vi "UpdateSelectedData.vi"(8 "error in (no error)":errorcluster, 9 "Old Value":i32, 11 "FakedArray in":refnum<class "FakedArray.lvclass">) -> (0 "error out":errorcluster, 3 "FakedArray out":refnum<class "FakedArray.lvclass">)   [LabVIEW 2020, in "FakedArray.lvclass"]
uses:
  FakedArray.lvclass
  FakedArray.lvclass/FakedArray.ctl
  vi.lib/LabVIEW Icon API/lv_icon/Controls/IEColor.ctl
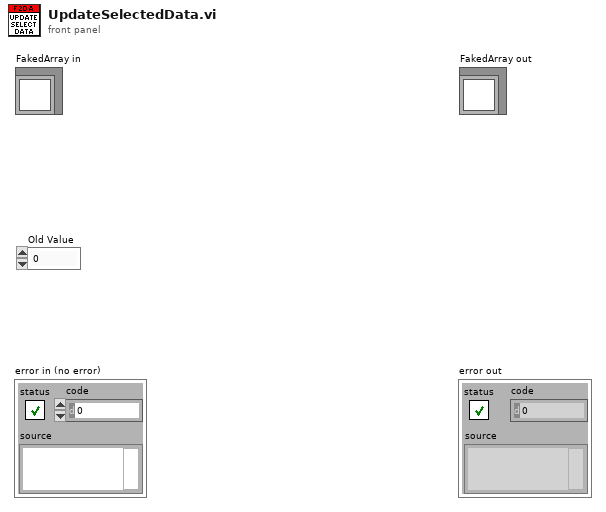
[diagram p1: front panel]
types:
  T1 = typedef "IEColor.ctl" = u32
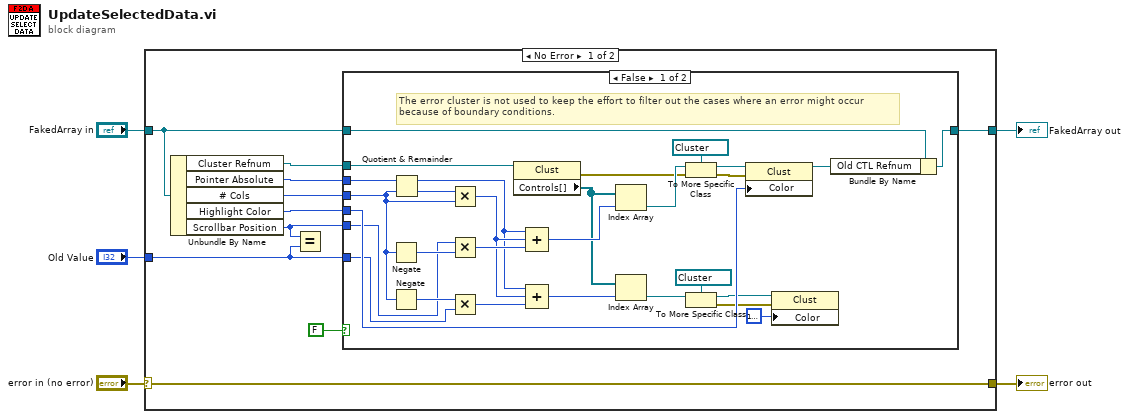
[diagram p0: block diagram]
diagram:
  n1 = case shown="No Error" "error in (no error)" {
    selector: "error in (no error)" -> [w7 w47]
    tunnel: [w7 w47] -> w4
    tunnel: [w10 w46] -> w2
    tunnel: "FakedArray in" -> [w15 w46]
    tunnel: "Old Value" -> [w8 _]
    frame No Error {
      n2 = Unbundle By Name(w15) -> ("Cluster Refnum"=w13:refnum<vi>, "Pointer Absolute"=w14:i32, "# Cols"=w11:i32, "Highlight Color"=w12:T1, "Scrollbar Position"=w9:i32)
      n3 = Equal?(x=w9, y=w8) -> ()  [unwired: 1 out]
      n4 = case shown="False" FALSE {
        tunnel: w15 -> [w44 w45]
        tunnel: w14 -> [w43 _]
        tunnel: w13 -> [w41 _]
        tunnel: w12 -> [w35 _]
        tunnel: w11 -> [w30 _]
        tunnel: [w19 w45] -> w10
        tunnel: w9 -> [w17 _]
        tunnel: w8 -> [w16 _]
        frame False {
          # "The error cluster is not used to keep the effort to filter out the cases where an error might occur\nbecause of boundary conditions."
          n5 = Negate(x=w30) -> (-x=w31:i32)
          n6 = Negate(x=w30) -> (-x=w32:i32)
          n7 = Quotient & Remainder(x=w43, y=w30) -> (x-y*floor(x/y)=w27:i32, floor(x/y)=w42:i32)
          n8 = Multiply(x=w42, y=w30) -> (x*y=w28:i32)
          n9 = Multiply(x=w17, y=w31) -> (x*y=w34:i32)
          n10 = Multiply(x=w32, y=w16) -> (x*y=w29:i32)
          n11 = property class="Clust"(reference=w41) -> (error out=w38:errorcluster, "Controls[]"=w26:refnum<vi>[])  [unwired: 1 in, 1 out]
          n12 = Compound Arithmetic op=ADD(w27, w28, w34) -> (w33:i32)
          n13 = Compound Arithmetic op=ADD(w27, w28, w29) -> (w25:i32)
          n14 = Index Array(array=w26, index=w33) -> (element=w39:refnum<vi>)
          n15 = Index Array(array=w26, index=w25) -> (element=w21:refnum<vi>)
          n16 = To More Specific Class(target class=refnum<vi> refnum ("Clust Refnum"), reference=w39, error in=w38) -> (specific class reference=w36:refnum<vi>, error out=w37:errorcluster)
          n17 = To More Specific Class(target class=refnum<vi> refnum ("Clust Refnum"), reference=w21) -> (specific class reference=w24:refnum<vi>, error out=w23:errorcluster)  [unwired: 1 in]
          n18 = property class="Clust"(reference=w36, error in=w37, "Color"=w35) -> (reference out=w18:refnum<vi>)  [unwired: 1 out]
          n19 = property class="Clust"(reference=w24, error in=w23, "Color"=T1 16777216 ("Highlight Color")) -> ()  [unwired: 2 out]
          n20 = Bundle By Name(cluster=w44, "Old CTL Refnum"=w18) -> (w19:refnum<class "FakedArray.lvclass">)
        }
        frame True {
        }
      }
    }
    frame Error {
    }
  }
  "error out" <- w4
  "FakedArray out" <- w2
